vi "Decompose LabVIEW Object - Aggregate - Private Data Cluster Value.vi"() -> ()   [LabVIEW 2017, in "Composition.Tests.lvlib"]
uses:
  Composition.Tests.lvlib
  Composition/Composition.lvlib
  Classes/Aggregate/Aggregate.lvclass
  Classes/String/String.lvclass
  Classes/Child/Child.lvclass
  <vilib>/addons/_JKI Toolkits/Caraya/classes/Test/Test.lvclass
  <vilib>/addons/_JKI Toolkits/Caraya/classes/Assert/Assert.lvclass
panel:
  out "error out":errorcluster
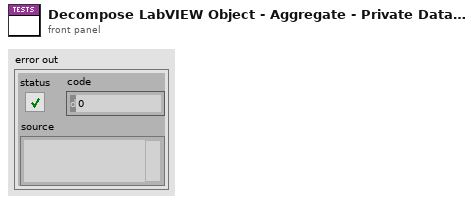
[diagram p1: front panel]
types:
  T1 = cluster{"String out":refnum<class "String.lvclass">, "Child out":refnum<class "Child.lvclass">}
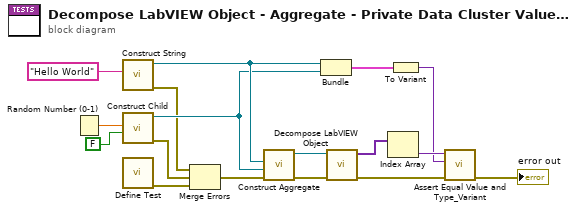
[diagram p0: block diagram]
diagram:
  n1 = Random Number (0-1)() -> (number: 0 to 1=w8:dbl)
  n2 = call "Construct String.vi"("String"="Hello World") -> ("error out"=w5:errorcluster, "String out"=w11:refnum<class "String.lvclass">)  [unwired: 9 in]
  n3 = call "Construct Child.vi"("Ignored"=FALSE, "Offset"=w8) -> ("error out"=w4:errorcluster, "Child out"=w9:refnum<class "Child.lvclass">)  [unwired: 8 in]
  n4 = call <vilib>:"Define Test.vi"() -> ("error out"=w3:errorcluster)  [unwired: 11 in]
  n5 = Merge Errors(w5, w4, w3) -> (w6:errorcluster)
  n6 = call "Construct Aggregate.vi"("error in (no error)"=w6, "Reflection.Tests.lvlib:Child.lvclass"=w9, "Reflection.Tests.lvlib:String.lvclass"=w11) -> ("error out"=w13:errorcluster, "Aggregate out"=w14:refnum<class "Aggregate.lvclass">)  [unwired: 7 in]
  n7 = Bundle("String out"=w11, "Child out"=w9) -> (w12:T1)  [unwired: 1 in]
  n8 = call "Decompose LabVIEW Object.vi"("error in (no error)"=w13, "LabVIEW Object"=w14) -> ("error out"=w17:errorcluster, "Private Data Clusters"=w15:variant[])  [unwired: 6 in, 2 out]
  n9 = Index Array(array=w15) -> (element=w2:variant)  [unwired: 1 in]
  n10 = To Variant(anything=w12) -> (Variant=w1:variant)
  n11 = call <vilib>:"Assert Equal Value and Type_Variant.vi"("error in (no error)"=w17, "Y"=w1, "X"=w2) -> ("error out"=→"error out":errorcluster)  [unwired: 8 in]
